vi "peak - calculate lorentzian.vi"(8 "4corners":T1={"z (-pi/2)"=-1.0311345636926572+0.5736824521422934i, "z(inf)"=-0.5200164984937075+1.0975277942502903i, "z (pi/2)"=-1.0311345636926572+0.5736824521422934i, "z center"=-0.5136528600391839+0.580046090596817i, "z(0)"=-0.5200164984937075+1.0975277942502903i, "radius"=-1.0311345636926572}, 9 "normalization factor":dbl, 10 "gamma":dbl, 11 "omega":dbl) -> (3 "lorentzian out":T2={"A (VHz)"=-1.0311345636926572, "ω (Hz)"=-1.0311345636926572, "Γ (Hz)"=-1.0311345636926572, "φ (rad)"=-1.0311345636926572, "Q"=-1.0311345636926572, "Norm  Ampl"=-1.0311345636926572, "z∞ (V)"=-1.0311345636926572+0.0i, "4corners"={"z (-pi/2)"=-1.0311345636926572+0.5736824521422934i, "z(inf)"=-0.5200164984937075+1.0975277942502903i, "z (pi/2)"=-1.0311345636926572+0.5736824521422934i, "z center"=-0.5136528600391839+0.580046090596817i, "z(0)"=-0.5200164984937075+1.0975277942502903i, "radius"=-1.0311345636926572}} {"z∞ (V)" format="%#_4p"; "Q" format="%#_4p"; "φ (rad)" format="%#_3p"; "Γ (Hz)" format="%#_5p"; "ω (Hz)" format="%#_9p"; "A (VHz)" format="%#_3p"})   [LabVIEW 2021]
uses:
  lorentzian.ctl
  circle corners.ctl
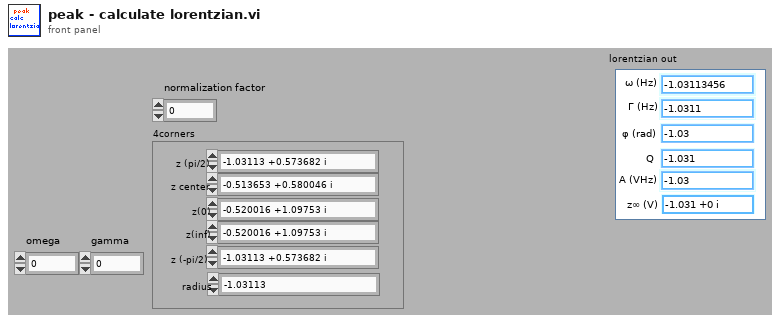
[diagram p1: front panel]
types:
  T1 = typedef "circle corners.ctl" = cluster{"z (-pi/2)":cdb, "z(inf)":cdb, "z (pi/2)":cdb, "z center":cdb, "z(0)":cdb, "radius":dbl}
  T2 = typedef "lorentzian.ctl" = cluster{"A (VHz)":dbl, "ω (Hz)":dbl, "Γ (Hz)":dbl, "φ (rad)":dbl, "Q":dbl, "Norm  Ampl":dbl, "z∞ (V)":cdb, "4corners":T1}
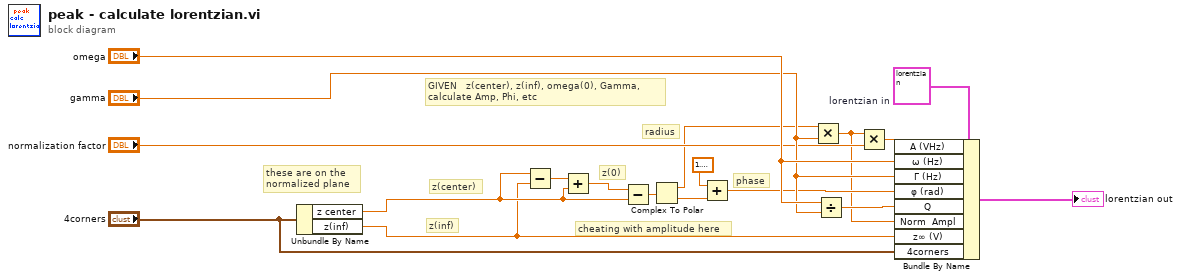
[diagram p0: block diagram]
diagram:
  w13 = T2 {"A (VHz)"=0.0, "ω (Hz)"=0.0, "Γ (Hz)"=0.0, "φ (rad)"=0.0, "Q"=0.0, "Norm  Ampl"=0.0, "z∞ (V)"=0.0+0.0i, "4corners"={"z (-pi/2)"=0.0+0.0i, "z(inf)"=0.0+0.0i, "z (pi/2)"=0.0+0.0i, "z center"=0.0+0.0i, "z(0)"=0.0+0.0i, "radius"=0.0}}  # lorentzian in
  # "these are on the \nnormalized plane"
  # "GIVEN   z(center), z(inf), omega(0), Gamma, \ncalculate Amp, Phi, etc"
  # "z(center)"
  # "z(0)"
  # "z(inf)"
  # "radius"
  # "phase"
  # "cheating with amplitude here"
  n1 = Unbundle By Name("4corners") -> ("z center"=w12:cdb, "z(inf)"=w11:cdb)
  n2 = Subtract(x=w12, y=w11) -> (x-y=w2:cdb)
  n3 = Add(x=w2, y=w12) -> (x+y=w1:cdb)
  n4 = Subtract(x=w1, y=w12) -> (x-y=w10:cdb)
  n5 = Complex To Polar(r * e^(i*theta)=w10) -> (r=w3:dbl, theta=w8:dbl)
  n6 = Add(x=1.5707963267948966, y=w8) -> (x+y=w7:dbl)
  n7 = Multiply(x=w3, y="gamma") -> (x*y=w5:dbl)
  n8 = Divide(x="omega", y="gamma") -> (x/y=w6:dbl)
  n9 = Multiply(x=w5, y="normalization factor") -> (x*y=w4:dbl)
  n10 = Bundle By Name(cluster=w13, "A (VHz)"=w4, "ω (Hz)"="omega", "Γ (Hz)"="gamma", "φ (rad)"=w7, "Q"=w6, "Norm  Ampl"=w5, "z∞ (V)"=w11, "4corners"="4corners") -> (→"lorentzian out":T2)
